vi "PromptForAttributes.vi"(9 "Attributes In":string[][](array[string]), 10 "Mouse Coords":T1, 11 "New Node Name":string) -> (2 "Canceled":bool, 3 "Attributes":string[][](array[string]))   [LabVIEW 2018]
uses:
  <vilib>/Utility/miscctls.llb/LVPoint32TypeDef.ctl
  Utils/FilePath.vi
  <vilib>/Utility/Data Type/NI_Data Type.lvlib
panel:
  out "Array":variant[](array[variant])
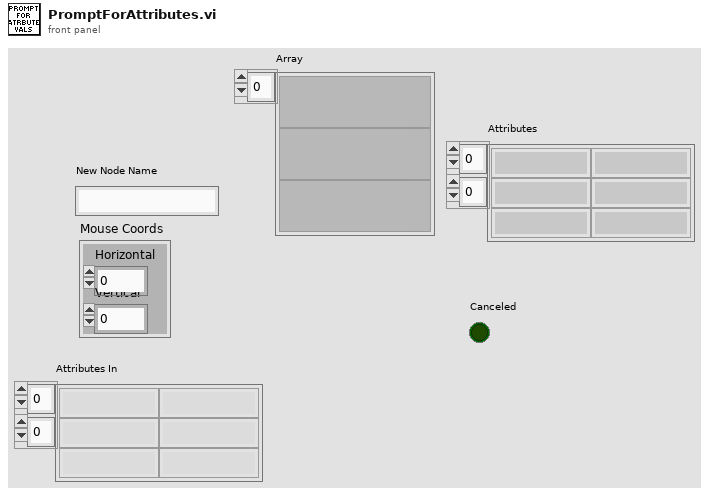
[diagram p1: front panel]
types:
  T1 = typedef "LVPoint32TypeDef.ctl" = cluster{"Horizontal":i32, "Vertical":i32}
  T2 = cluster{"Horizontal":i32, "Vertical":i32, "Horizontal":i32, "Vertical":i32}
  T3 = typedef "NI_Data Type.lvlib/Data Type.ctl" = enum8{"Invalid Type", "Void", "I8", "I16", "I32", "I64", "U8", "U16", "U32", "U64", "Single Float", "Double Float", "Extended Float", "Single Complex", "Double Complex", "Extended Complex", "Enum U8", "Enum U16", "Enum U32", "Enum U64", "Single Float With Unit", "Double Float With Unit", "Extended Float With Unit", "Single Complex with Unit", "Double Complex with Unit", "Extended Complex with Unit", "Boolean", "String", "Path", "Picture", "Tag", "Array", "Cluster", "Variant", "LV Variant", "Waveform", "Timestamp", "Digital Waveform", "Digital Data", "ExpressData", "Refnum", "External Data", "VI", "Poly VI", "LabVIEW Class Instance", "Fixed Point"}
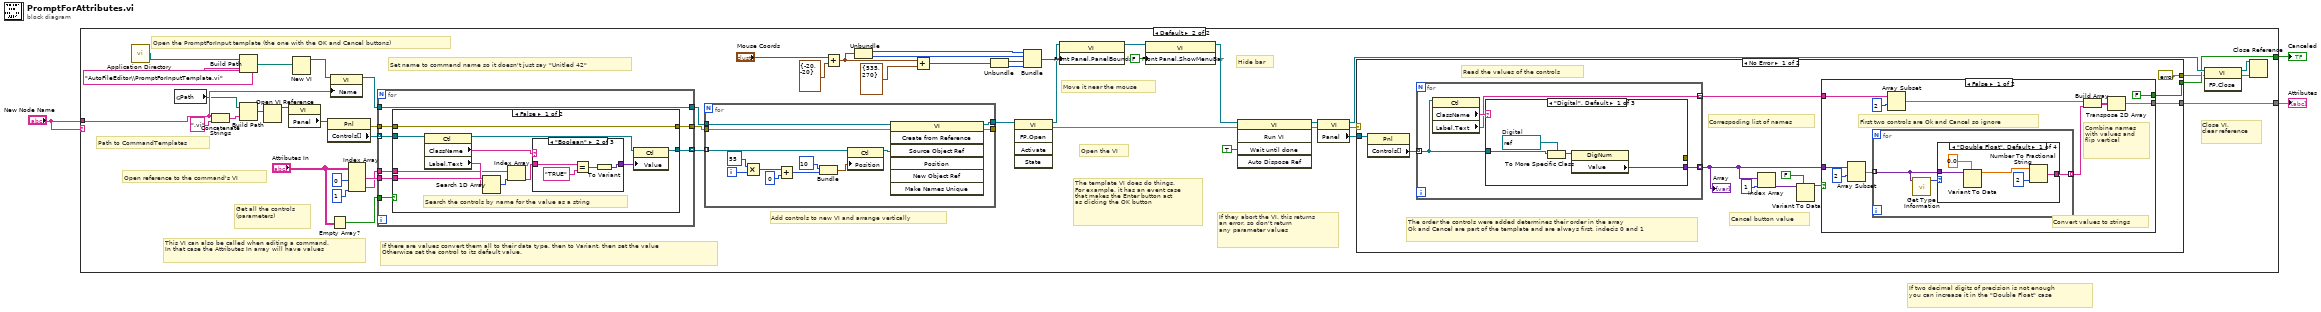
[diagram p0: block diagram]
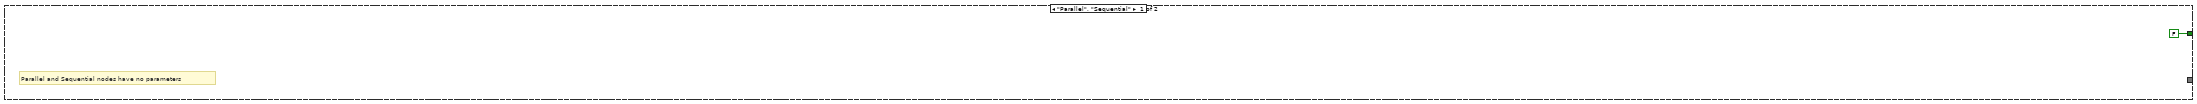
[diagram p2: hidden frame]
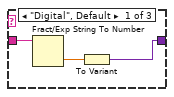
[diagram p3: hidden frame]
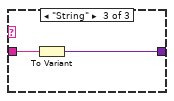
[diagram p4: hidden frame]
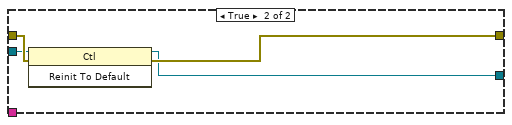
[diagram p5: hidden frame]
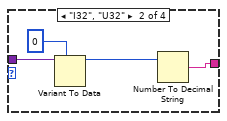
[diagram p6: hidden frame]
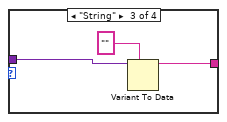
[diagram p7: hidden frame]
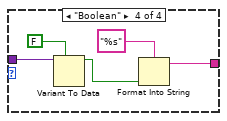
[diagram p8: hidden frame]
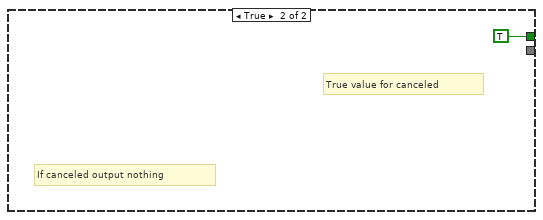
[diagram p9: hidden frame]
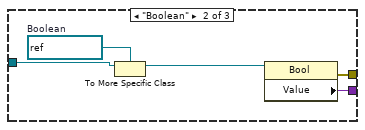
[diagram p10: hidden frame]
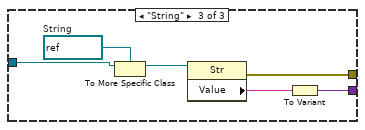
[diagram p11: hidden frame]
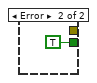
[diagram p12: hidden frame]
diagram:
  # "If two decimal digits of precision is not enough\nyou can increase it in the \"Double Float\" case"
  n1 = case shown="Default" "New Node Name" {
    tunnel: "New Node Name" -> [_ w10]
    tunnel: [FALSE ("Canceled") w40] -> w3
    tunnel: [_ w39] -> w2
    frame "Parallel", "Sequential" {
      # "Parallel and Sequential nodes have no parameters"
    }
    frame Default {
      # "The template VI does do things.\nFor example, it has an event case\nthat makes the Enter button act\nas clicking the OK button"
      # "Hide bar"
      # "Close VI,\nclear reference"
      # "If there are values convert them all to their data type, then to Variant, then set the value\nOtherwise set the control to its default value."
      # "This VI can also be called when editing a command.\nIn that case the Attributes In array will have values"
      # "Set name to command name so it doesn't just say \"Unitled 42\""
      # "Open the VI"
      # "Get all the controls\n(parameters)"
      # "Path to CommandTemplates"
      # "If they abort the VI, this returns\nan error, so don't return\nany parameter values"
      # "Open reference to the command's VI"
      # "Move it near the mouse"
      # "Add controls to new VI and arrange vertically"
      # "Open the PromptForInput template (the one with the OK and Cancel buttons)"
      n2 = call <vilib>:"Application Directory.vi"() -> ("Application Directory"=w8:path)
      n3 = global read "FilePath.vi" "Path"() -> (w9:path)
      n4 = Concatenate Strings(w10, ".vi" ("string")) -> (w43:string)
      n5 = Build Path(base path=w8, name or relative path="AutoFileEditor\\PromptForInputTemplate.vi") -> (appended path=w45:path)
      n6 = Build Path(base path=w9, name or relative path=w43) -> (appended path=w42:path)
      n7 = Open VI Reference(vi path=w42) -> (vi reference=w24:refnum<vi>)  [unwired: 5 in, 1 out]
      n8 = property class="VI"(reference=w24) -> ("Panel"=w54:refnum<vi>)  [unwired: 1 in, 2 out]
      n9 = New VI(10:w45) -> (3:w49:refnum<vi>)  [unwired: 6 in, 1 out]
      n10 = property class="Pnl"(reference=w54) -> (error out=w18:errorcluster, "Controls[]"=w21:refnum<vi>[])  [unwired: 1 in, 1 out]
      n11 = property class="VI"(reference=w49, "Name"=w10) -> (reference out=w17:refnum<vi>)  [unwired: 1 in, 1 out]
      n12 = Empty Array?(array="Attributes In") -> (empty?=w11:bool)
      n13 = Index Array(array="Attributes In", index (col) #1=0 ("disabled index (col)"), index (col) #2=1 ("index (col)")) -> (element #1=w15:string[], element #2=w13:string[])  [unwired: 2 in]
      n14 = for {
        tunnel: w21 -> [w60] mode=indexing
        tunnel: [w61] -> w20 mode=indexing
        tunnel: [w55] -> w19
        tunnel: w18 -> [w56]
        tunnel: [w62] -> w5
        tunnel: w17 -> [w62]
        tunnel: w15 -> [w59]
        tunnel: w13 -> [w58]
        tunnel: w11 -> [w57]
        n15 = case shown="False" w57 {
          tunnel: [w64 w84] -> w61
          tunnel: w60 -> [w73 w83]
          tunnel: w59 -> [w71 _]
          tunnel: w58 -> [w69 _]
          tunnel: w56 -> [w65 w86]
          tunnel: [w65 w85] -> w55
          frame False {
            # "Search the controls by name for the value as a string"
            n16 = property class="Ctl"(reference=w73) -> (reference out=w63:refnum<vi>, "ClassName"=w72:string, "Label.Text"=w70:string)  [unwired: 1 in, 1 out]
            n17 = Search 1D Array(1D array=w71, element=w70) -> (index of element=w68:i32)  [unwired: 1 in]
            n18 = Index Array(array=w69, index=w68) -> (element=w67:string)
            n19 = case shown="\"Boolean\"" w72 {
              tunnel: w67 -> [w76 w80 w82]
              tunnel: [w74 w77 w81] -> w66
              frame "Digital", Default {
                n20 = Fract/Exp String To Number(string=w76) -> (number=w75:dbl)  [unwired: 3 in, 1 out]
                n21 = To Variant(anything=w75) -> (Variant=w74:variant)
              }
              frame "Boolean" {
                n22 = Equal?(x=w80, y="TRUE") -> (x = y?=w78:bool)
                n23 = To Variant(anything=w78) -> (Variant=w77:variant)
              }
              frame "String" {
                n24 = To Variant(anything=w82) -> (Variant=w81:variant)
              }
            }
            n25 = property class="Ctl"(reference=w63, "Value"=w66) -> (reference out=w64:refnum<vi>)  [unwired: 1 in, 1 out]
          }
          frame True {
            n26 = invoke class="Ctl" method="Reinit To Default"(reference=w83, error in=w86) -> (reference out=w84:refnum<vi>, error out=w85:errorcluster)  [unwired: 1 in, 1 out]
          }
        }
      }
      n27 = for {
        tunnel: w19 -> [w161]
        tunnel: w20 -> [w151] mode=indexing
        tunnel: [w160] -> w22
        tunnel: [w159] -> _
        tunnel: w5 -> [w149]
        i -> [w158]
        n28 = Multiply(x=55, y=w158) -> (x*y=w156:i32)
        n29 = Add(x=w156, y=0) -> (x+y=w153:i32)
        n30 = Bundle("y"=10, w153) -> (w150:cluster{"y":i32, i32})  [unwired: 1 in]
        n31 = property class="Ctl"(reference=w151, "Position"=w150) -> (reference out=w154:refnum<vi>)  [unwired: 1 in, 1 out]
        n32 = invoke class="VI" method="Create from Reference"(reference=w149, error in=w161, "Source Object Ref"=w154) -> (reference out=w160:refnum<vi>, error out=w159:errorcluster)  [unwired: 4 in, 5 out]
      }
      n33 = Add(x="Mouse Coords", y=T1 {"Horizontal"=-20, "Vertical"=-20}) -> (x+y=w26:T1)
      n34 = Unbundle(w26) -> ("Horizontal"=w33:i32, "Vertical"=w32:i32)
      n35 = Add(x=w26, y=cluster{"Left":i16, "Top":i16} {"Left"=535, "Top"=270} ("Front Panel Window:Panel Bounds")) -> (x+y=w35:T1)
      n36 = Unbundle(w35) -> ("Horizontal"=w31:i32, "Vertical"=w30:i32)
      n37 = invoke class="VI" method="FP.Open"(reference=w22) -> (reference out=w6:refnum<vi>, error out=w48:errorcluster)  [unwired: 4 in, 3 out]
      n38 = Bundle("Horizontal"=w33, "Vertical"=w32, "Horizontal"=w31, "Vertical"=w30) -> (w29:T2)  [unwired: 1 in]
      n39 = property class="VI"(reference=w6, "Front Panel.PanelBounds"=w29) -> (reference out=w23:refnum<vi>)  [unwired: 1 in, 1 out]
      n40 = property class="VI"(reference=w23, "Front Panel.ShowMenuBar"=FALSE ("Front Panel Window:Show Menu Bar")) -> (reference out=w7:refnum<vi>)  [unwired: 1 in, 1 out]
      n41 = invoke class="VI" method="Run VI"(reference=w7, error in=w48, "Wait until done"=TRUE ("Wait Until Done")) -> (reference out=w50:refnum<vi>, error out=w51:errorcluster)  [unwired: 2 in, 3 out]
      n42 = property class="VI"(reference=w50, error in=w51) -> (reference out=w53:refnum<vi>, error out=w41:errorcluster, "Panel"=w52:refnum<vi>)
      n43 = case shown="No Error" w41 {
        tunnel: w52 -> [w96 _]
        tunnel: [w92 TRUE ("Canceled")] -> w40
        tunnel: [w89 _] -> w39
        tunnel: [errorcluster {"status"=FALSE, "code"=0, "source"=""} ("error constant") _] -> w36
        frame No Error {
          # "The order the controls were added determines their order in the array\nOk and Cancel are part of the template and are always first, indecis 0 and 1"
          # "Correspoding list of names"
          # "Cancel button value"
          # "Read the values of the controls"
          n44 = property class="Pnl"(reference=w96) -> ("Controls[]"=w97:refnum<vi>[])  [unwired: 1 in, 2 out]
          n45 = for {
            tunnel: w97 -> [w132] mode=indexing
            tunnel: [w130] -> w91 mode=indexing
            tunnel: [w129] -> w88 mode=indexing
            n46 = property class="Ctl"(reference=w132) -> ("ClassName"=w131:string, "Label.Text"=w129:string)  [unwired: 1 in, 2 out]
            n47 = case shown="\"Digital\", Default" w131 {
              tunnel: [_ w139 w145] -> _
              tunnel: w132 -> [w134 w138 w144]
              tunnel: [w133 w137 w142] -> w130
              frame "Digital", Default {
                w136 = refnum<vi> refnum  # Digital
                n48 = To More Specific Class(target class=w136, reference=w134) -> (specific class reference=w135:refnum<vi>)  [unwired: 1 in, 1 out]
                n49 = property class="DigNum"(reference=w135) -> ("Value"=w133:variant)  [unwired: 1 in, 2 out]
              }
              frame "Boolean" {
                w141 = refnum<vi> refnum  # Boolean
                n50 = To More Specific Class(target class=w141, reference=w138) -> (specific class reference=w140:refnum<vi>)  [unwired: 1 in, 1 out]
                n51 = property class="Bool"(reference=w140) -> (error out=w139:errorcluster, "Value"=w137:variant)  [unwired: 1 in, 1 out]
              }
              frame "String" {
                w147 = refnum<vi> refnum  # String
                n52 = To More Specific Class(target class=w147, reference=w144) -> (specific class reference=w146:refnum<vi>)  [unwired: 1 in, 1 out]
                n53 = property class="Str"(reference=w146) -> (error out=w145:errorcluster, "Value"=w143:string)  [unwired: 1 in, 1 out]
                n54 = To Variant(anything=w143) -> (Variant=w142:variant)
              }
            }
          }
          "Array" <- w91
          n55 = Index Array(array=w91, index=1) -> (element=w95:variant)
          n56 = Variant To Data(type=FALSE, Variant=w95) -> (data=w93:bool)  [unwired: 1 in, 1 out]
          n57 = case shown="False" w93 {
            tunnel: [FALSE ("Wait Until Done") TRUE ("Wait Until Done")] -> w92
            tunnel: w91 -> [w106 _]
            tunnel: [w98 _] -> w89
            tunnel: w88 -> [w101 _]
            frame False {
              # "Combine names\nwith values and\nflip vertical"
              # "First two controls are Ok and Cancel so ignore"
              # "Convert values to strings"
              n58 = Array Subset(array=w106, index=2) -> (w104:variant[])  [unwired: 1 in]
              n59 = for {
                tunnel: w104 -> [w109] mode=indexing
                tunnel: [w108] -> w103 mode=indexing
                n60 = call <vilib>:"Get Type Information.vi"("Variant"=w109) -> ("Type"=w110:T3)  [unwired: 6 in, 4 out]
                n61 = case shown="\"Double Float\", Default" w110 {
                  tunnel: w109 -> [w113 w118 w122 w127]
                  tunnel: [w111 w117 w120 w125] -> w108
                  frame "Double Float", Default {
                    n62 = Variant To Data(type=0.0, Variant=w113) -> (data=w115:dbl)  [unwired: 1 in, 1 out]
                    n63 = Number To Fractional String(number=w115, precision (6)=i16 2) -> (F-format string=w111:string)  [unwired: 2 in]
                  }
                  frame "I32", "U32" {
                    n64 = Variant To Data(type=i16 0 ("precision (6)"), Variant=w118) -> (data=w119:i16)  [unwired: 1 in, 1 out]
                    n65 = Number To Decimal String(number=w119) -> (decimal integer string=w117:string)  [unwired: 1 in]
                  }
                  frame "String" {
                    n66 = Variant To Data(type="", Variant=w122) -> (data=w120:string)  [unwired: 1 in, 1 out]
                  }
                  frame "Boolean" {
                    n67 = Variant To Data(type=FALSE ("Wait Until Done"), Variant=w127) -> (data=w123:bool)  [unwired: 1 in, 1 out]
                    n68 = Format Into String(format string="%s", w123) -> (resulting string=w125:string)  [unwired: 2 in, 1 out]
                  }
                }
              }
              n69 = Array Subset(array=w101, index=2) -> (w100:string[])  [unwired: 1 in]
              n70 = Build Array(w100, w103) -> (w99:string[][])
              n71 = Transpose 2D Array(2D array=w99) -> (transposed array=w98:string[][])
            }
            frame True {
              # "True value for canceled"
              # "If canceled output nothing"
            }
          }
        }
        frame Error {
        }
      }
      n72 = invoke class="VI" method="FP.Close"(reference=w53, error in=w36) -> (reference out=w38:refnum<vi>, error out=w37:errorcluster)  [unwired: 1 in, 1 out]
      n73 = Close Reference(reference=w38, error in (no error)=w37) -> ()  [unwired: 1 out]
    }
  }
  "Attributes" <- w2
  "Canceled" <- w3
